vi "saveAsDocument.vi"(8 "error in (no error)":errorcluster, 10 "File Path":path, 11 "MS-Excel in":refnum<class "MS-Excel.lvclass">) -> (0 "error out":errorcluster, 3 "MS-Excel out":refnum<class "MS-Excel.lvclass">)   [LabVIEW 2020, in "LabVIEW NPOI.lvlib" / "MS-Excel.lvclass"]
uses:
  MS-Excel.lvclass
  MS-Excel.lvclass/MS-Excel.ctl
  D:/Benjamin/Documents/Perso/Code/WC/LabVIEW_NPOI/lib/NPOI 2.1.1/NPOI.dll
  lib/NPOI 2.1.1/NPOI.dll
  Support/File Stream/File Stream.lvlib
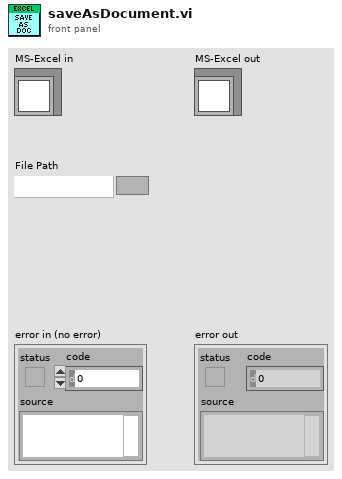
[diagram p1: front panel]
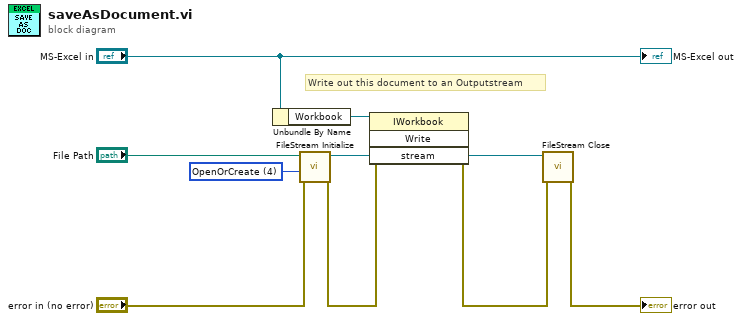
[diagram p0: block diagram]
diagram:
  w6 = 4 items=["CreateNew"=1, "Create"=2, "Open"=3, "OpenOrCreate"=4, "Truncate"=5, "Append"=6] ("operation")
  # "Write out this document to an Outputstream"
  n1 = Unbundle By Name("MS-Excel in") -> ("Workbook"=w8:refnum<k24>)
  n2 = call "FileStream Initialize.vi"("error in (no error)"="error in (no error)", "mode"=w6, "path"="File Path") -> ("error out"=w5:errorcluster, "new reference"=w3:refnum<k24>)  [unwired: 7 in]
  n3 = invoke class="IWorkbook" method="Write"(reference=w8, error in=w5, "stream"=w3) -> (error out=w2:errorcluster)  [unwired: 1 in, 3 out]
  n4 = call "FileStream Close.vi"("error in (no error)"=w2, "reference"=w3) -> ("error out"=→"error out":errorcluster)  [unwired: 9 in]
  "MS-Excel out" <- "MS-Excel in"
